vi "Temp Setting Display.vi"(7 "JL LEDs":T1) -> (8 "Temp Setting":i32)   [LabVIEW 2016]
uses:
  type defs/UI_LEDs.ctl
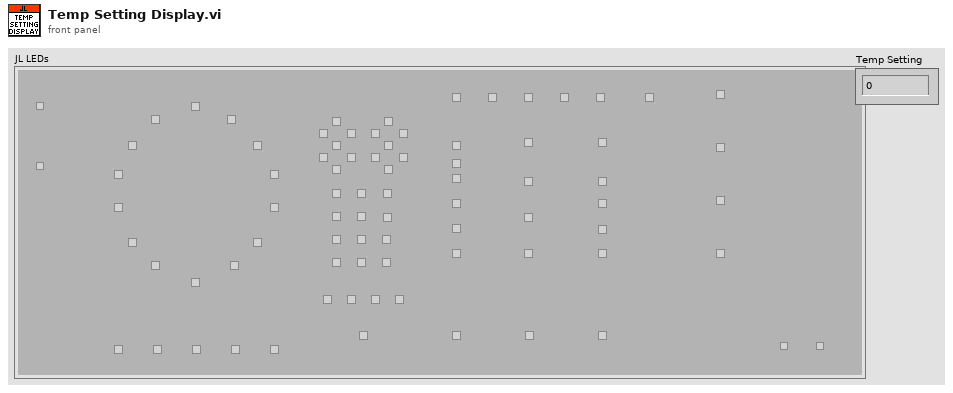
[diagram p1: front panel]
types:
  T1 = typedef "UI_LEDs.ctl" = cluster{"Z301 - Encoder 0":bool, "Z302 - Encoder 13":bool, "Z303 - Encoder 12":bool, "Z304 - Encoder 11":bool, "Z305 - Encoder 10":bool, "Z306 - Encoder 09":bool, "Z307 - Encoder 08":bool, "Z308 - Encoder 07":bool, "Z309 - Encoder 06":bool, "Z310 - Encoder 05":bool, "Z311 - Encoder 04":bool, "Z312 - Encoder 03":bool, "Z313 - Encoder 02":bool, "Z314 - Encoder 01":bool, "Z315 - Unpopulated":bool, "Z316 - Unpopulated":bool, "Z317 - SSD1:A":bool, "Z318 - SSD1:B":bool, "Z319 - SSD1:G":bool, "Z320 - SSD1:C":bool, "Z321 - SSD1:D":bool, "Z322 - SSD1:E":bool, "Z323 - SSD1:F":bool, "Z324 - Pause 1":bool, "Z325 - Control Lock 1":bool, "Z326 - Sensing 1":bool, "Z327 - Clean Lint Filter 1":bool, "Z328 - Extra Status 1":bool, "Z329 - Extra Status 2":bool, "Z330 - Clean Lint Filter 2":bool, "Z331 -Sensing 2":bool, "Z332 - Unpopulated":bool, "Z333 - SSD2:A":bool, "Z334 - SSD2:B":bool, "Z335 - SSD2:G":bool, "Z345 - SSD2:C":bool, "Z336 - SSD2:D":bool, "Z337 - SSD2:E":bool, "Z338 - SSD2:F":bool, "Z339 - Pause 3":bool, "Z340 - Control Lock 3":bool, "Z353 - Sensing 3":bool, "Z342 - Clean Lint Filter 3":bool, "Z344 - Extra Status 3":bool, "Z346 - Extra Status 4":bool, "Z341 - Pause 2":bool, "Z343 - Control Lock 2":bool, "Z347 - Unpopulated":bool, "Z348 -My Cycle":bool, "Z349 - Delay Dry":bool, "Z350 - Volume":bool, "Z351 - Damp Alert":bool, "Z352 - Bar 1":bool, "Z354 - Bar 2":bool, "Z355 - Bar 3":bool, "Z356 - Bar 4":bool, "Z357 - Bar 5":bool, "Z358 - eDry":bool, "Z359 - Time Increment":bool, "Z360 - Time Decrement":bool, "Z361 - Extended Tumble":bool, "Z362 - Unpopulated":bool, "Z363 - Unpopulated":bool, "Z364 - Unpopulated":bool, "Z365 - Status 1":bool, "Z366 - Status 3":bool, "Z367 - Default Time 5":bool, "Z368 - Default Time 4":bool, "Z369 - Default Time 3":bool, "Z370 - Dry":bool, "Z371 - Status 2":bool, "Z372 -Default Time 2":bool, "Z373 - Default Time 1":bool, "Z374 - Unpopulated":bool, "Z375 - Default Time 0":bool, "Z376 - No Heat":bool, "Z377 - Unpopulated":bool, "Z378 - Unpopulated":bool, "Z379 - Unpopulated":bool, "Z380 - Unpopulated":bool, "Z381 - Status 4":bool, "Z382 - Status 6":bool, "Z383 - More Dry":bool, "Z384 - High":bool, "Z385 - Medium":bool, "Z386 -Low":bool, "Z387 - Status 5":bool, "Z388 - Less Dry":bool, "Z388 - Extra Low":bool, "Z390 - Unpopulated":bool, "Z391 - Damp":bool, "Z392 - Unpopulated":bool, "Z393 - Unpopulated":bool, "Z394 - Unpopulated":bool, "Z395 - Unpopulated":bool, "Z396 - Unpopulated":bool, "Z101 - unpop?":bool, "Z102 - Start/Pause":bool, "OFF - OFF":bool, "MAX - MAX":bool}
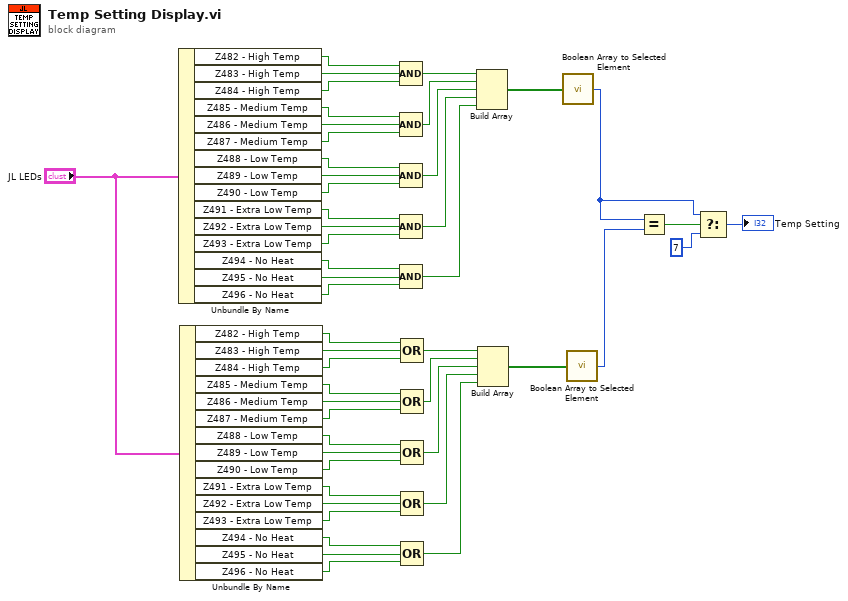
[diagram p0: block diagram]
diagram:
  n1 = Unbundle By Name("JL LEDs") -> ("Z482 - High Temp"=w48:bool, "Z483 - High Temp"=w47:bool, "Z484 - High Temp"=w46:bool, "Z485 - Medium Temp"=w44:bool, "Z486 - Medium Temp"=w43:bool, "Z487 - Medium Temp"=w42:bool, "Z488 - Low Temp"=w41:bool, "Z489 - Low Temp"=w40:bool, "Z490 - Low Temp"=w39:bool, "Z491 - Extra Low Temp"=w37:bool, "Z492 - Extra Low Temp"=w38:bool, "Z493 - Extra Low Temp"=w36:bool, "Z494 - No Heat"=w34:bool, "Z495 - No Heat"=w35:bool, "Z496 - No Heat"=w33:bool)
  n2 = Unbundle By Name("JL LEDs") -> ("Z482 - High Temp"=w28:bool, "Z483 - High Temp"=w27:bool, "Z484 - High Temp"=w26:bool, "Z485 - Medium Temp"=w24:bool, "Z486 - Medium Temp"=w23:bool, "Z487 - Medium Temp"=w22:bool, "Z488 - Low Temp"=w21:bool, "Z489 - Low Temp"=w20:bool, "Z490 - Low Temp"=w19:bool, "Z491 - Extra Low Temp"=w17:bool, "Z492 - Extra Low Temp"=w18:bool, "Z493 - Extra Low Temp"=w16:bool, "Z494 - No Heat"=w14:bool, "Z495 - No Heat"=w15:bool, "Z496 - No Heat"=w13:bool)
  n3 = Compound Arithmetic op=AND(w48, w47, w46) -> (w45:bool)
  n4 = Compound Arithmetic op=AND(w44, w43, w42) -> (w32:bool)
  n5 = Compound Arithmetic op=AND(w41, w40, w39) -> (w31:bool)
  n6 = Compound Arithmetic op=AND(w37, w38, w36) -> (w30:bool)
  n7 = Compound Arithmetic op=AND(w34, w35, w33) -> (w29:bool)
  n8 = Compound Arithmetic op=OR(w28, w27, w26) -> (w25:bool)
  n9 = Compound Arithmetic op=OR(w24, w23, w22) -> (w12:bool)
  n10 = Compound Arithmetic op=OR(w21, w20, w19) -> (w11:bool)
  n11 = Compound Arithmetic op=OR(w17, w18, w16) -> (w10:bool)
  n12 = Compound Arithmetic op=OR(w14, w15, w13) -> (w9:bool)
  n13 = Build Array(w45, w32, w31, w30, w29) -> (w8:bool[])
  n14 = Build Array(w25, w12, w11, w10, w9) -> (w7:bool[])
  n15 = call "Boolean Array to Selected Element.vi"("Bool Array In"=w8) -> ("Selected Element Out"=w4:i32)  [unwired: 14 in]
  n16 = call "Boolean Array to Selected Element.vi"("Bool Array In"=w7) -> ("Selected Element Out"=w5:i32)  [unwired: 14 in]
  n17 = Equal?(x=w4, y=w5) -> (x = y?=w6:bool)
  n18 = Select(t=w4, s=w6, f=7) -> (s? t:f=→"Temp Setting":i32)
